vi "CMN_GetLineNumber.vi"(6 "line no":i32=-1, 10 "multi-line string":string="gress 185 of 270\rprogress 185 of 270\rprogress 185 of 270\rprogress 185 of 270\rprogress 185 of 270\rprogress 185 of 270\rprogress 185 of 270\rprogress 185 of 270\rprogress 185 of 270\rprogress 185 of 270\rprogress 185 of 270\rprogress 185 of 270\rprogress 185 of 270\rprogress 185 of 270\rprogress 185 of 270\rprogress 185 of 270\rprogress 185 of 270\rprogress 185 of 270\rprogress 185 of 270\rprogress 185 of 270\rprogress 185 of 270\rprogress 185 of 270\rprogress 185 of 270\rprogress 185 of 270\rprogress 185 of 270\rprogress 185 of 270\rprogress 185 of 270\rprogress 185 of 270\rprogress 185 of 270\rprogress 185 of 270\rprogress 185 of 270\rprogress 185 of 270\rprogress 185 of 270\rprogress 185 of 270\rprogress 185 of 270\rprogress 185 of 270\rERROR system is busy (reading)\n") -> (2 "line":string)   [LabVIEW 2016]
panel:
  # "index 1: first line, 2: second line, ...  (beginign to end)\nindex -1: last line, -2: second last line, .. (end to begining)"
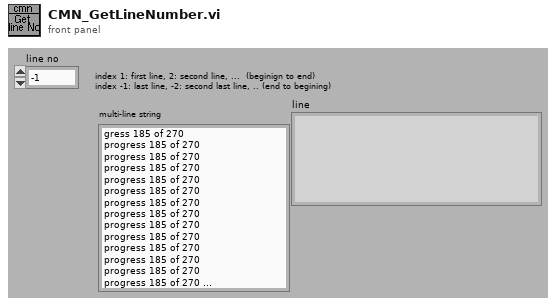
[diagram p1: front panel]
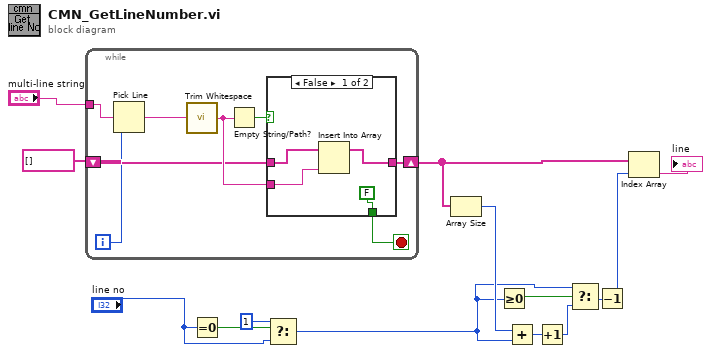
[diagram p0: block diagram]
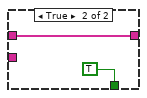
[diagram p2: hidden frame]
diagram:
  n1 = while {
    shift-right: [w20] -> w14
    shift-left: string[] [] -> [w19]
    tunnel: "multi-line string" -> [w15]
    i -> [w18]
    stop <- w16 stop-if-true
    n2 = Pick Line(multi-line string=w15, line index=w18) -> (output string=w17:string)  [unwired: 1 out]
    n3 = call <vilib>:"Trim Whitespace.vi"("string"=w17) -> ("trimmed string"=w21:string)  [unwired: 1 in]
    n4 = Empty String/Path?(string/path=w21) -> (empty?=w22:bool)
    n5 = case shown="False" w22 {
      tunnel: w21 -> [w26 _]
      tunnel: [w25 w28] -> w20
      tunnel: w19 -> [w24 w28]
      tunnel: [FALSE TRUE] -> w16
      frame False {
        n6 = Insert Into Array(array=w24, new element=w26) -> (w25:string[])  [unwired: 1 in]
      }
      frame True {
      }
    }
  }
  n7 = Equal To 0?(x="line no") -> (x = 0?=w11:bool)
  n8 = Select(t=1, s=w11, f="line no") -> (s? t:f=w5:i32)
  n9 = Array Size(array=w14) -> (size(s)=w6:i32)
  n10 = Greater Or Equal To 0?(x=w5) -> (x >= 0?=w13:bool)
  n11 = Add(x=w6, y=w5) -> (x+y=w4:i32)
  n12 = Increment(x=w4) -> (x+1=w3:i32)
  n13 = Select(t=w5, s=w13, f=w3) -> (s? t:f=w8:i32)
  n14 = Decrement(x=w8) -> (x-1=w7:i32)
  n15 = Index Array(array=w14, index=w7) -> (element=→"line":string)
